vi "Is Control Present.vi"(8 "Error In":errorcluster, 10 "Control label":string, 11 "VI ref":refnum<vi>) -> (0 "Error Out":errorcluster, 1 "Ctl Refnum":refnum<vi>, 2 "Present":bool, 3 "VI ref out":refnum<vi>)   [LabVIEW 2019]
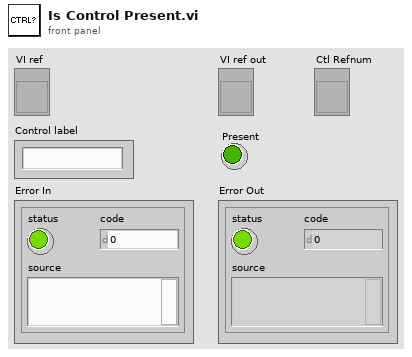
[diagram p1: front panel]
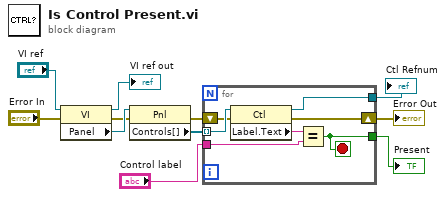
[diagram p0: block diagram]
diagram:
  n1 = property class="VI"(reference="VI ref", error in="Error In") -> (reference out=→"VI ref out":refnum<vi>, error out=w7:errorcluster, "Panel"=w10:refnum<vi>)
  n2 = property class="Pnl"(reference=w10, error in=w7) -> (error out=w6:errorcluster, "Controls[]"=w9:refnum<vi>[])  [unwired: 1 out]
  n3 = for {
    tunnel: w9 -> [w18] mode=indexing
    shift-right: [w16] -> w4
    shift-left: w6 -> [w17]
    tunnel: "Control label" -> [w14]
    tunnel: [w12] -> w3
    tunnel: [w13] -> w1
    stop <- w12 stop-if-true
    n4 = property class="Ctl"(reference=w18, error in=w17) -> (reference out=w13:refnum<vi>, error out=w16:errorcluster, "Label.Text"=w15:string)
    n5 = Equal?(x=w15, y=w14) -> (x = y?=w12:bool)
  }
  "Error Out" <- w4
  "Present" <- w3
  "Ctl Refnum" <- w1
